vi "ReadExperimentRunsNode.vi"(8 "Error In":errorcluster, 11 "Experiment Node In":refnum<k20>) -> (0 "Error Out":errorcluster, 2 "Experiment Runs":T1[](array[typedef]), 3 "Experiment Node Out":refnum<k20>)   [LabVIEW 2012]
uses:
  ExperimentRun.ctl
  ExperimentRunTiming.ctl
  ExperimentRunDose.ctl
  ExperimentRunFluence.ctl
  ExperimentRunTotalCharge.ctl
  <vilib>/xml/NI_XML.lvlib
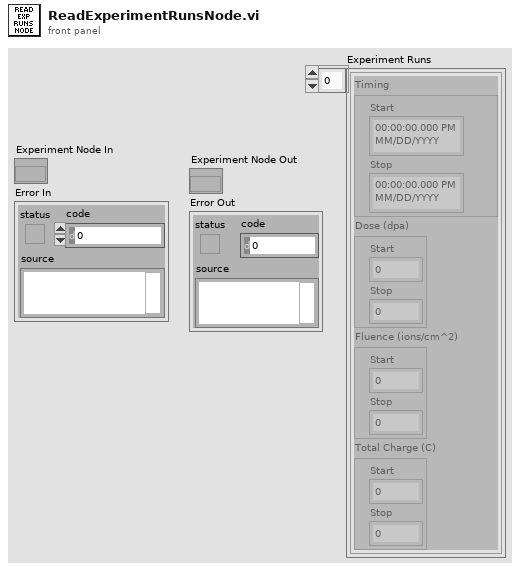
[diagram p1: front panel]
types:
  T1 = typedef "ExperimentRun.ctl" = cluster{"Timing":T2, "Dose (dpa)":T3, "Fluence (ions/cm^2)":T4, "Total Charge (C)":T5}
  T2 = typedef "ExperimentRunTiming.ctl" = cluster{"Start":timestamp, "Stop":timestamp}
  T3 = typedef "ExperimentRunDose.ctl" = cluster{"Start":dbl, "Stop":dbl}
  T4 = typedef "ExperimentRunFluence.ctl" = cluster{"Start":dbl, "Stop":dbl}
  T5 = typedef "ExperimentRunTotalCharge.ctl" = cluster{"Start":dbl, "Stop":dbl}
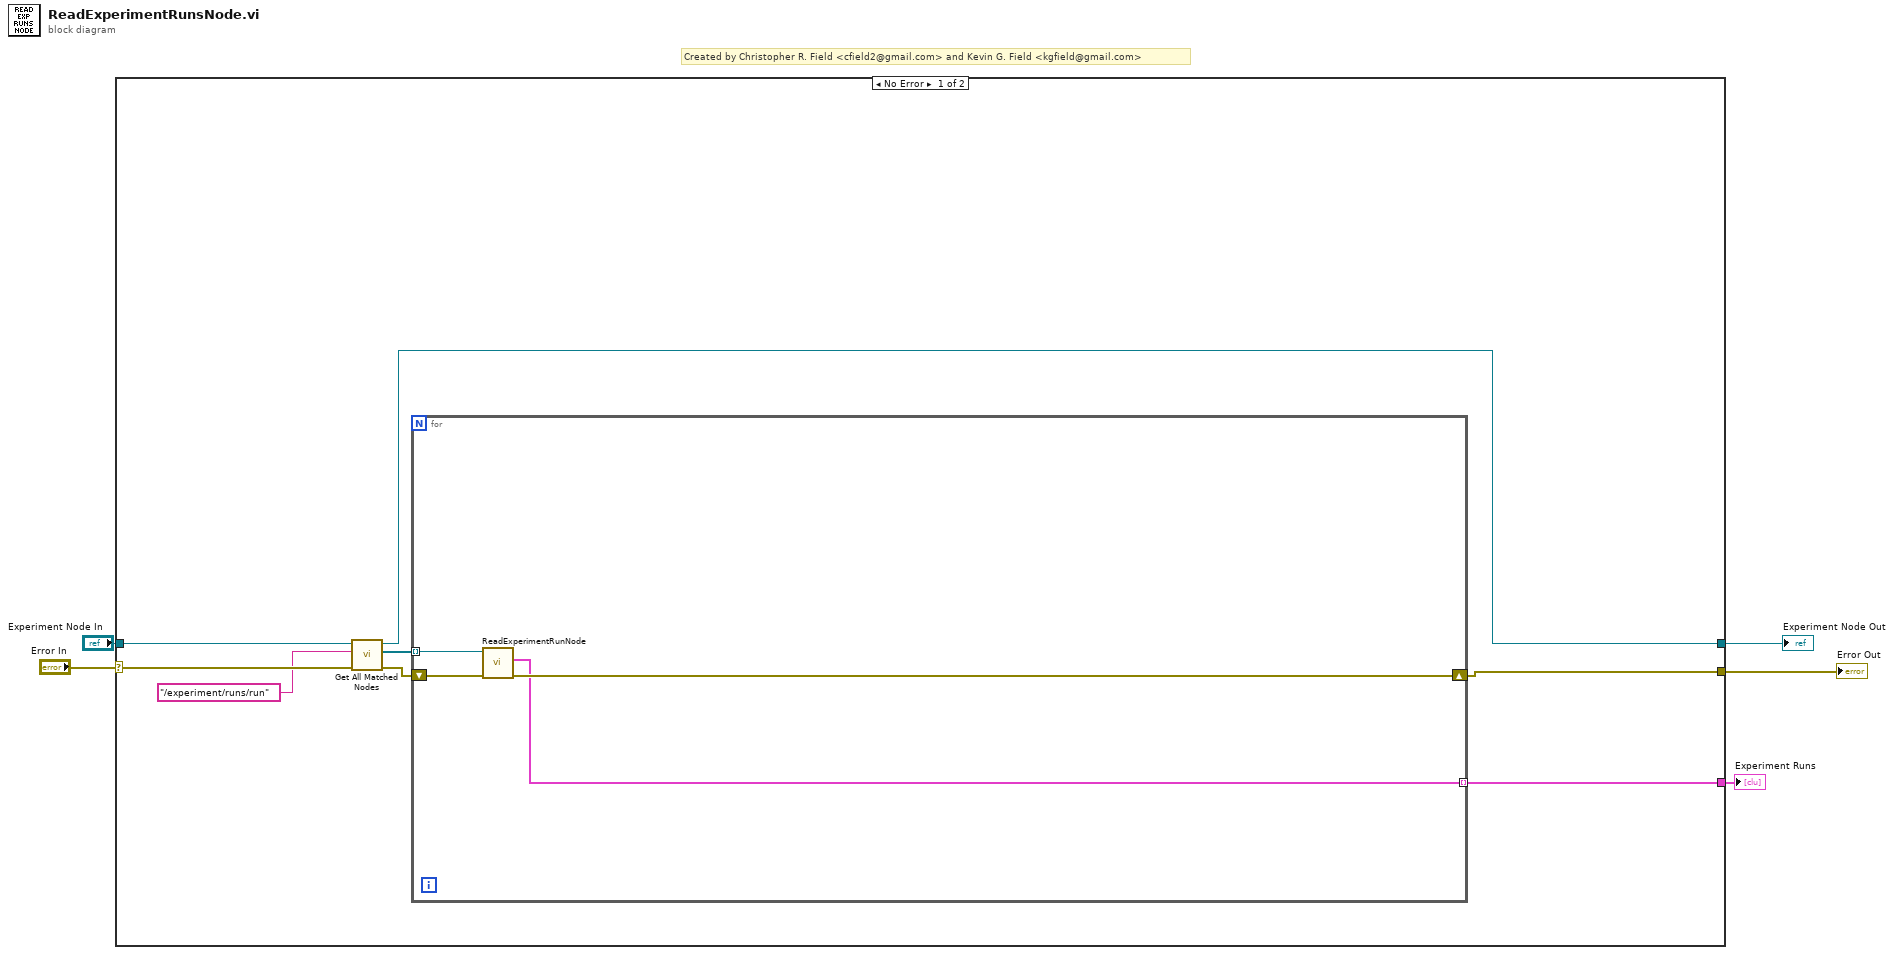
[diagram p0: block diagram]
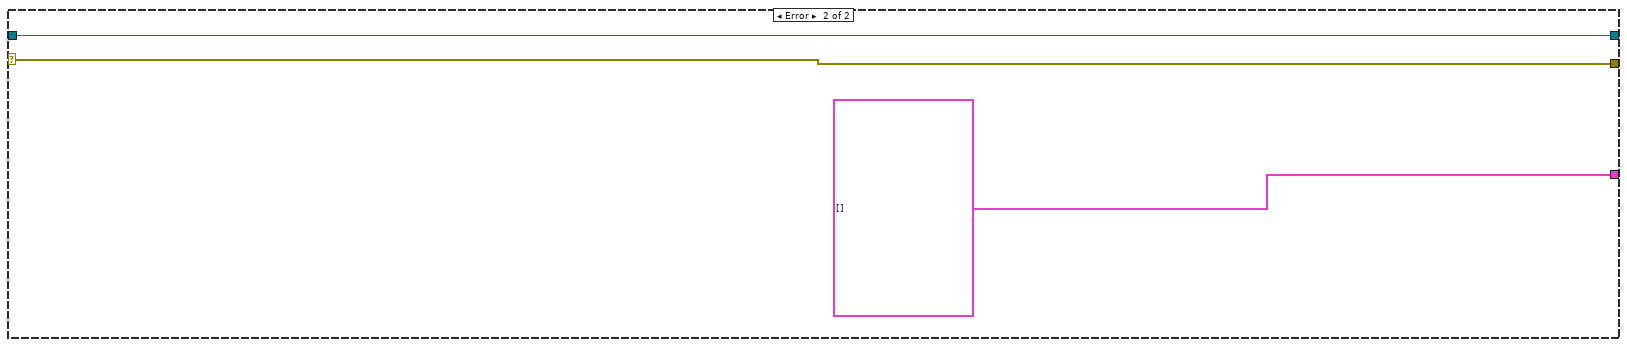
[diagram p2: hidden frame]
diagram:
  # "Created by Christopher R. Field <cfield2@gmail.com> and Kevin G. Field <kgfield@gmail.com>"
  n1 = case shown="No Error" "Error In" {
    selector: "Error In" -> [w12 w19]
    tunnel: "Experiment Node In" -> [w13 w20]
    tunnel: [w8 w20] -> w3
    tunnel: [w7 w19] -> w2
    tunnel: [w6 T1[] []] -> w1
    frame No Error {
      n2 = call <vilib>:"Get All Matched Nodes.vi"("error in (no error)"=w12, "XPath expression"="/experiment/runs/run", "node in"=w13) -> ("error out"=w9:errorcluster, "node result array"=w10:refnum<k20>[], "node out"=w8:refnum<k20>)  [unwired: 6 in]
      n3 = for {
        tunnel: w10 -> [w17] mode=indexing
        shift-right: [w15] -> w7
        shift-left: w9 -> [w16]
        tunnel: [w14] -> w6 mode=indexing
        n4 = call "ReadExperimentRunNode.vi"("Error In"=w16, "Experiment Run Node In"=w17) -> ("Error Out"=w15:errorcluster, "Experiment Run"=w14:T1)  [unwired: 7 in, 1 out]
      }
    }
    frame Error {
    }
  }
  "Experiment Node Out" <- w3
  "Error Out" <- w2
  "Experiment Runs" <- w1
